vi "ClustersAndJson.vi"() -> ()   [LabVIEW 2013]
uses:
  <vilib>/addons/JSON API/JSON Object/JSON Object.lvclass
  <vilib>/addons/JSON API/JSON Object/Set Object Item by name.vi
  <vilib>/addons/JSON API/JSON Scalar/Set String.vi
  <vilib>/addons/JSON API/JSON Value/Get as JSON string (pretty).vi
  <vilib>/addons/JSON API/Get Polymorphic/JSON GetSet.lvlib
  <vilib>/addons/JSON API/JSON Value/JSON Value.lvclass
  <vilib>/addons/JSON API/JSON Scalar/JSON Scalar.lvclass
panel:
  out "String":string
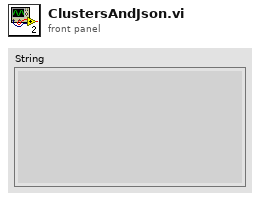
[diagram p1: front panel]
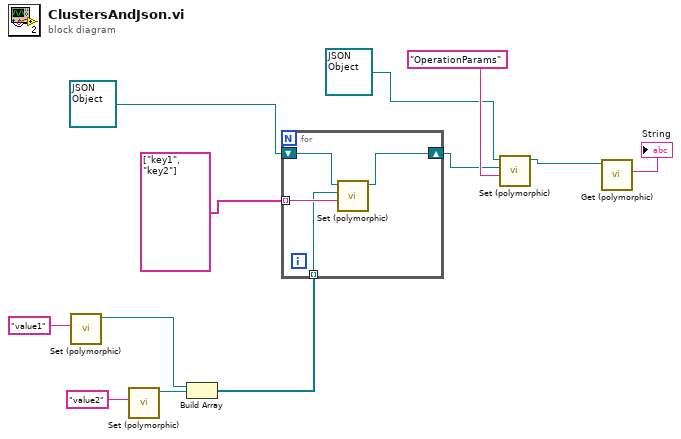
[diagram p0: block diagram]
diagram:
  n1 = call-poly <vilib>:"Set (polymorphic).vi"("String"="value1") -> ("JSON Scalar out"=w8:refnum<class "JSON Scalar.lvclass">)  [unwired: 9 in, 1 out]
  n2 = call-poly <vilib>:"Set (polymorphic).vi"("String"="value2") -> ("JSON Scalar out"=w10:refnum<class "JSON Scalar.lvclass">)  [unwired: 9 in, 1 out]
  n3 = Build Array(w8, w10) -> (w7:refnum<class "JSON Scalar.lvclass">[])
  n4 = for {
    tunnel: string[] ["key1", "key2"] -> [w16] mode=indexing
    tunnel: w7 -> [w15] mode=indexing
    shift-right: [w13] -> w2
    shift-left: refnum<class "JSON Object.lvclass"> refnum ("JSON Object in") -> [w14]
    n5 = call-poly <vilib>:"Set (polymorphic).vi"("name"=w16, "Value"=w15, "JSON Object in"=w14) -> ("JSON Object out"=w13:refnum<class "JSON Object.lvclass">)  [unwired: 6 in, 2 out]
  }
  n6 = call-poly <vilib>:"Set (polymorphic).vi"("name"="OperationParams", "Value"=w2, "JSON Object in"=refnum<class "JSON Object.lvclass"> refnum) -> ("JSON Object out"=w4:refnum<class "JSON Object.lvclass">)  [unwired: 6 in, 2 out]
  n7 = call-poly <vilib>:"Get (polymorphic).vi"("JSON Value in"=w4) -> ("String"=→"String":string)  [unwired: 9 in, 1 out]
